vi "Run Measurement Remotely on Client.vi"(4 "Show UI?":bool, 6 "Array of Devices":string[](array[string]), 8 "error in (no error)":errorcluster, 9 "Measurement Name":string, 10 "ConnectionID":string, 11 "Server Controller in":refnum<class "Server Controller.lvclass">) -> (0 "error out":errorcluster, 3 "Server Controller out":refnum<class "Server Controller.lvclass">)   [LabVIEW 2026, in "Server Controller.lvlib" / "Server Controller.lvclass"]
uses:
  Server Controller.lvclass
  C:/Users/E2013170/Documents/GitHub/Measurement-Utility-Reference/source/framework/Controller/Controller.lvclass
  framework/Controller/Messages/Launch Measurements Message/Launch Measurements Message.lvclass
  C:/Program Files/National Instruments/LabVIEW 2026/vi.lib/ActorFramework/Message/Message.lvclass
  framework/Controller/Messages/Launch Measurements Message/Launch Measurements Message.lvclass/Launch Measurements Message.ctl
  framework/Measurement Actor/Measurement.lvclass
  recovery/packages/ni_lib_linked_network_actor-1.2.0.19-9492AF5A82/File Group 0/vi.lib/NI/Actors/Linked Network Actor/Linked Network Actor Messages/Transmit Network Message Msg/Transmit Network Message Msg.lvclass
  framework/Controller/Controller.lvclass
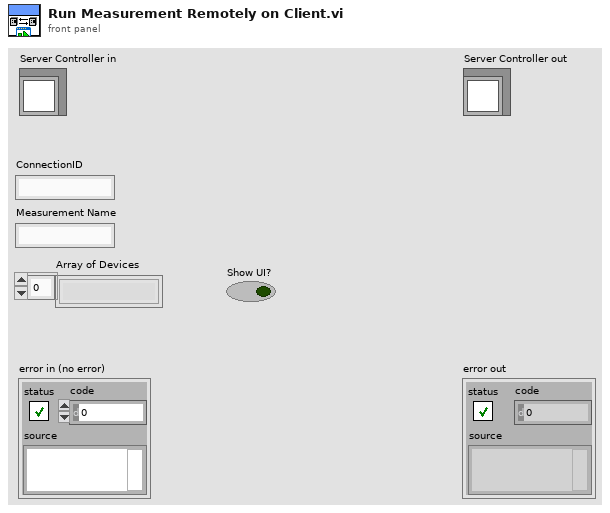
[diagram p1: front panel]
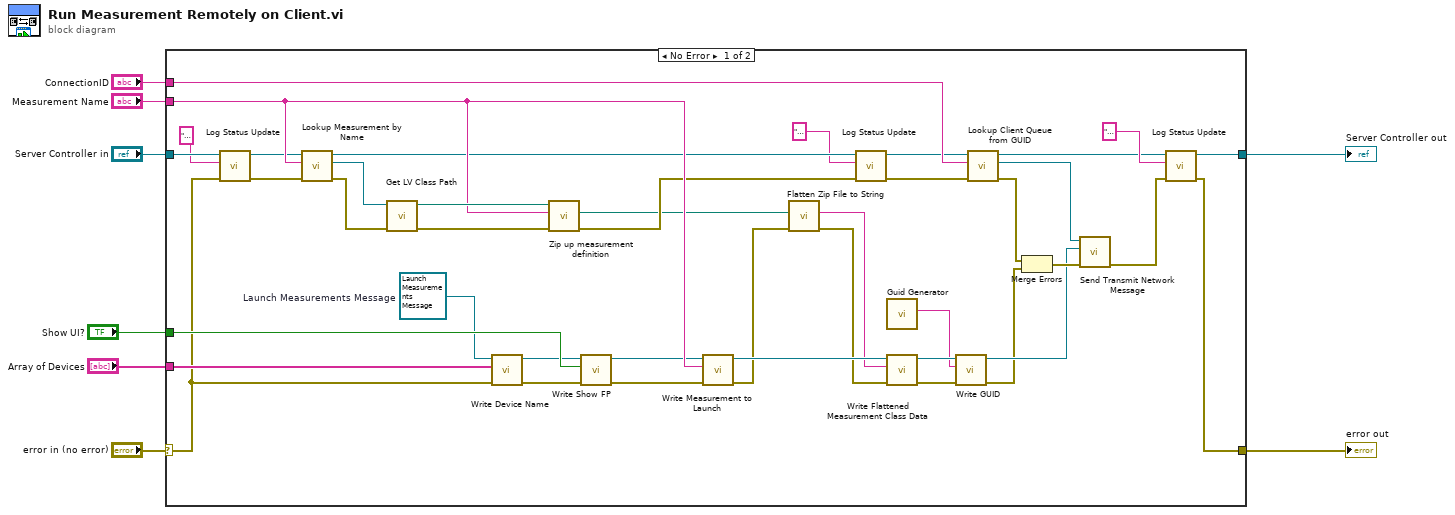
[diagram p0: block diagram]
diagram:
  n1 = case shown="No Error" "error in (no error)" {
    selector: "error in (no error)" -> [w31 w50]
    tunnel: [w19 w50] -> w7
    tunnel: [w21 w49] -> w5
    tunnel: "Server Controller in" -> [w33 w49]
    tunnel: "ConnectionID" -> [w48 _]
    tunnel: "Measurement Name" -> [w42 _]
    tunnel: "Array of Devices" -> [w46 _]
    tunnel: "Show UI?" -> [w45 _]
    frame No Error {
      w40 = refnum<class "Launch Measurements Message.lvclass"> refnum  # Launch Measurements Message
      n2 = call-dynamic "Log Status Update.vi"("error in (no error)"=w31, "String"="Preparing to Upload Measurement", "Controller in"=w33) -> ("error out"=w30:errorcluster, "Controller out"=w32:refnum<class "Server Controller.lvclass">)  [unwired: 7 in]
      n3 = call "Lookup Measurement by Name.vi"("error in (no error)"=w30, "Measurement Name"=w42, "Controller in"=w32) -> ("error out"=w25:errorcluster, "Measurement.lvclass"=w44:refnum<class "Measurement.lvclass">, "Controller out"=w28:refnum<class "Server Controller.lvclass">)  [unwired: 5 in, 1 out]
      n4 = call <vilib>:"Get LV Class Path.vi"("error in (no error)"=w25, "object"=w44) -> ("error out"=w41:errorcluster, "class path"=w43:path)  [unwired: 8 in]
      n5 = call "Write Device Name.vi"("error in (no error)"=w31, "Device Names"=w46, "Launch Measurements Message in"=w40) -> ("error out"=w37:errorcluster, "Launch Measurements Message out"=w39:refnum<class "Launch Measurements Message.lvclass">)  [unwired: 7 in]
      n6 = call "Zip up measurement definition.vi"("error in (no error)"=w41, "Measurement Name"=w42, "class path"=w43) -> ("error out"=w24:errorcluster, "output path"=w14:path)  [unwired: 7 in]
      n7 = call "Write Show FP.vi"("error in (no error)"=w37, "Show FP?"=w45, "Launch Measurements Message in"=w39) -> ("error out"=w36:errorcluster, "Launch Measurements Message out"=w38:refnum<class "Launch Measurements Message.lvclass">)  [unwired: 7 in]
      n8 = call "Write Measurement to Launch.vi"("error in (no error)"=w36, "Measurement Name"=w42, "Launch Measurements Message in"=w38) -> ("error out"=w16:errorcluster, "Launch Measurements Message out"=w18:refnum<class "Launch Measurements Message.lvclass">)  [unwired: 7 in]
      n9 = call "Flatten Zip File to String.vi"("error in"=w16, "Path"=w14) -> ("error out"=w15:errorcluster, "String"=w13:string)  [unwired: 8 in]
      n10 = call-dynamic "Log Status Update.vi"("error in (no error)"=w24, "String"="Measurement uploaded to web server successfully", "Controller in"=w28) -> ("error out"=w23:errorcluster, "Controller out"=w27:refnum<class "Server Controller.lvclass">)  [unwired: 7 in]
      n11 = call "Guid Generator.vi"() -> ("GUID"=w11:string)  [unwired: 10 in, 1 out]
      n12 = call "Write Flattened Measurement Class Data.vi"("error in (no error)"=w15, "Flattened Measurement Class Data"=w13, "Launch Measurements Message in"=w18) -> ("error out"=w10:errorcluster, "Launch Measurements Message out"=w17:refnum<class "Launch Measurements Message.lvclass">)  [unwired: 7 in]
      n13 = call "Write GUID.vi"("error in (no error)"=w10, "GUID"=w11, "Launch Measurements Message in"=w17) -> ("error out"=w9:errorcluster, "Launch Measurements Message out"=w12:refnum<class "Launch Measurements Message.lvclass">)  [unwired: 7 in]
      n14 = call "Lookup Client Queue from GUID.vi"("error in (no error)"=w23, "GUID"=w48, "Server Controller in"=w27) -> ("error out"=w34:errorcluster, "Caller-To-Actor Enqueuer"=w47:refnum<class "Message Enqueuer.lvclass">, "Server Controller out"=w21:refnum<class "Server Controller.lvclass">)  [unwired: 5 in, 1 out]
      n15 = Merge Errors(w34, w9) -> (w35:errorcluster)
      n16 = call "Send Transmit Network Message.vi"("error in (no error)"=w35, "Message"=w12, "Message Enqueuer"=w47) -> ("error out"=w20:errorcluster)  [unwired: 7 in, 1 out]
      n17 = call-dynamic "Log Status Update.vi"("error in (no error)"=w20, "String"="Client instructed to run measurement", "Controller in"=w21) -> ("error out"=w19:errorcluster)  [unwired: 7 in, 1 out]
    }
    frame Error {
    }
  }
  "error out" <- w7
  "Server Controller out" <- w5
